vi "ReloadSession.vi"(8 "error in (no error)":errorcluster, 11 "session id in":i32) -> (0 "error out":errorcluster, 3 "session id out":i32)   [LabVIEW 2017, in "libonnx_wrapper.lvlib"]
doc: "/**\n * @brief Перезагрузить сессию по сохранённому пути\n * \n * Восстанавливает сессию после вызова UnloadSession. Модель загружается заново\n * из файла, путь к которому был сохранён при создании сессии.\n * \n * @param sessionId [IN] ID сессии для перезагрузки\n * \n * @return int32: 0 при успешной загрузке\n * @return int32: -1 если сессия не найдена или путь не сохранён\n * \n * @note Требует предварительного вызова CreateSession\n * @note Полезно для экономии памяти в долго работающих приложениях\n */\nint ReloadSession(int sessionId);"
uses:
  libonnx_wrapper.lvlib
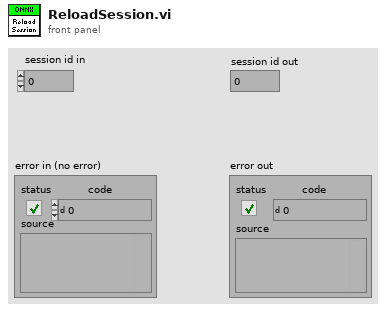
[diagram p1: front panel]
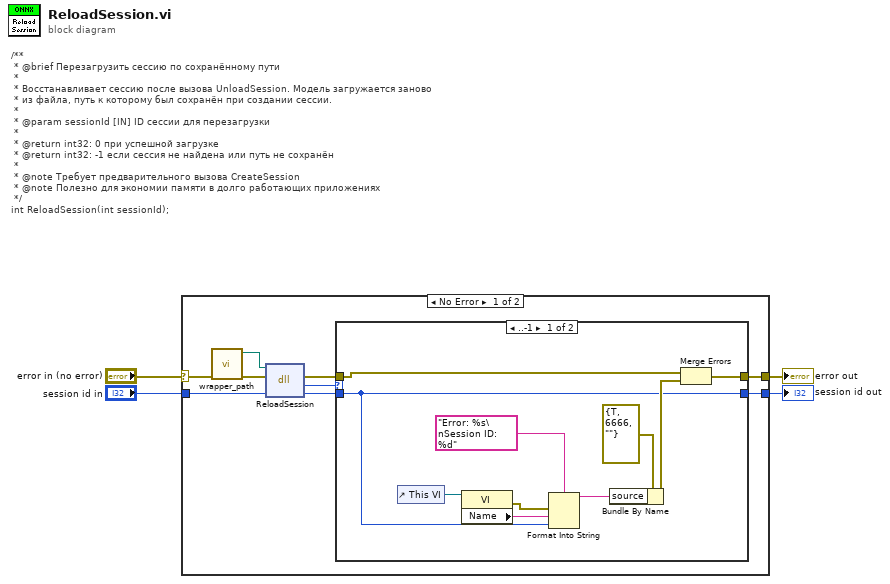
[diagram p0: block diagram]
diagram:
  # "/**\n * @brief Перезагрузить сессию по сохранённому пути\n * \n * Восстанавливает сессию после вызова UnloadSession. Модель загружается заново\n * из файла, путь к которому был сохранён при создании сессии.\n * \n * @param sessionId [IN] ID сессии для перезагрузки\n * \n * @return int32: 0 при успешной загрузке\n * @return int32: -1 если сессия не найдена или путь не сохранён\n * \n * @note Требует предварительного вызова CreateSession\n * @note Полезно для экономии памяти в долго работающих приложениях\n */\nint ReloadSession(int sessionId);"
  n1 = case shown="No Error" "error in (no error)" {
    selector: "error in (no error)" -> [w5 w27]
    tunnel: "session id in" -> [w11 w26]
    tunnel: [w9 w27] -> w3
    tunnel: [w6 w26] -> w2
    frame No Error {
      n2 = call "wrapper_path.vi"("error in (no error)"=w5) -> ("error out"=w13:errorcluster, "wrapper path"=w12:path)  [unwired: 9 in]
      n3 = dll-call lib="home/ivan/LabVIEWData/ONNX/Test/libonnx_wrapper/unix64/libonnx_wrapper.so" fn="ReloadSession"(path in=w12, error in=w13, "sessionId"=w11) -> (error out=w10:errorcluster, "return"=w8:i32, "sessionId"=w7:i32)  [unwired: 1 in, 1 out]
      n4 = case shown="..-1" w8 {
        tunnel: w10 -> [w14 w25]
        tunnel: [w15 w25] -> w9
        tunnel: w7 -> [w16 w24]
        tunnel: [w16 w24] -> w6
        frame ..-1 {
          n5 = control-ref of="This VI"() -> (w20:refnum<vi>)
          n6 = property class="VI"(reference=w20) -> (error out=w17:errorcluster, "Name"=w19:string)  [unwired: 1 in, 1 out]
          n7 = Format Into String(format string="Error: %s\nSession ID: %d", error in=w17, w19, w16) -> (resulting string=w21:string)  [unwired: 1 in, 1 out]
          n8 = Bundle By Name(cluster=errorcluster {"status"=TRUE, "code"=6666, "source"=""} ("error out"), "source"=w21) -> (w22:errorcluster)
          n9 = Merge Errors(w14, w22) -> (w15:errorcluster)
        }
        frame 0.. {
        }
      }
    }
    frame Error {
    }
  }
  "error out" <- w3
  "session id out" <- w2
